vi "ARC_Queue Create_Single.vi"(8 "error in":errorcluster caption="Error In (no error)", 10 "Max Queue Size(-1)":i32=-1, 11 "Queue Name":string) -> (0 "error out":errorcluster caption="Error Out", 2 "Created New?":bool, 3 "Queue Name dup":string)   [LabVIEW 2016]
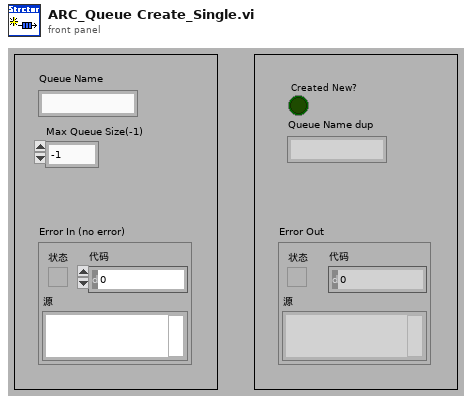
[diagram p1: front panel]
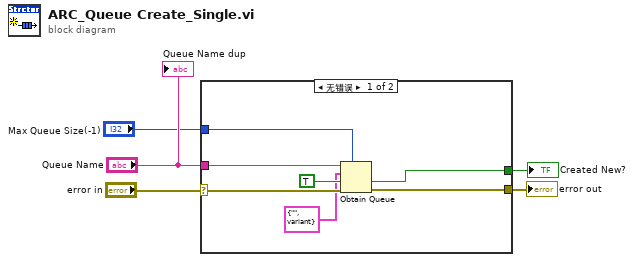
[diagram p0: block diagram]
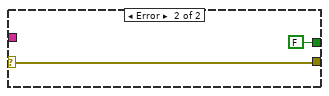
[diagram p2: hidden frame]
diagram:
  n1 = case shown="无错误" "error in" {
    selector: "error in" -> [w11 w14]
    tunnel: [w10 w14] -> w4
    tunnel: "Queue Name" -> [w9 _]
    tunnel: "Max Queue Size(-1)" -> [w8 _]
    tunnel: [w7 FALSE ("created new?")] -> w1
    frame No Error {
      n2 = Obtain Queue(max queue size (-1, unlimited)=w8, name (unnamed)=w9, element data type=cluster{"Event":string, "Data":variant} {"Event"="", "Data"=variant} ("输出簇"), create if not found? (T)=TRUE ("如未找到是否创建？(T)"), error in (no error)=w11) -> (created new?=w7:bool, error out=w10:errorcluster)  [unwired: 1 out]
    }
    frame Error {
    }
  }
  "error out" <- w4
  "Created New?" <- w1
  "Queue Name dup" <- "Queue Name"
